vi "ILC Cyber Learning.vi"(6 "PID Cluster":T4={"L1 to L4 PID Cluster"={"L1 PID Gains"={"Kp"=0.005, "Kd"=0.5, "Ki"=0.0005}, "L2 PID Gains"={"Kp"=0.01, "Kd"=1.0, "Ki"=0.005}, "L3 PID Gains"={"Kp"=0.05, "Kd"=1.0, "Ki"=0.0005}, "L4 PID Gains"={"Kp"=0.1, "Kd"=0.1, "Ki"=0.0005}}, "Stage PID Cluster"={"Stage Z PID"={"Kp"=0.0005, "Kd"=0.001, "Ki"=0.0}, "Stage Y PID"={"Kp"=0.0003, "Kd"=0.01, "Ki"=0.0}, "Stage X PID"={"Kp"=0.0003, "Kd"=0.01, "Ki"=0.0}}, "OCT Z PID Gains"={"Kp"=0.0003, "Kd"=0.0001, "Ki"=0.01}}, 7 "Input RUY":T1, 8 "error in":errorcluster, 9 "Offset Home 2 RCM":dbl[](array[numeric])=[0.0, 0.0, 0.0, 0.0], 10 "Prev Posit Cluster":T3={"Prev L1 to L4 Posit"=[-0.5319, -0.035669172703475985, -2.0566170657346783, 0.9099264705882353], "Prev Stage Posit"=[6.002553885707208, 5.996566124542428, 5.995469940427586], "Prev OCT Z Posit"=-0.0}, 11 "FPGA VI Reference In":refnum<k20>) -> (0 "error out":errorcluster, 2 "Last Posit Cluster":T2={"Last L1 to L4 Posit"=[0.0, 0.0, 0.0, 0.0], "Last Stage Posit"=[6.0, 6.0, 6.0], "Last OCT Z Posit"=0.0}, 3 "FPGA VI Reference Out":refnum<k20>, 5 "Updated RUY":T1)   [LabVIEW 2016]
uses:
  <vilib>/Platform/TimedLoop/XDataNode/timing_clust.ctl
  <vilib>/Platform/TimedLoop/XDataNode/nitl_modes.ctl
  <vilib>/Platform/TimedLoop/XDataNode/wakeup.ctl
  Global Variables.vi
  <vilib>/platform/TimedLoop/XDataNode/XDataNode.xnode
  <vilib>/Platform/TimedLoop/XDataNode/XDNodeRunTimeDep.lvlib
panel:
  out "In Servo Loop":bool
  out "Loading Finished":bool
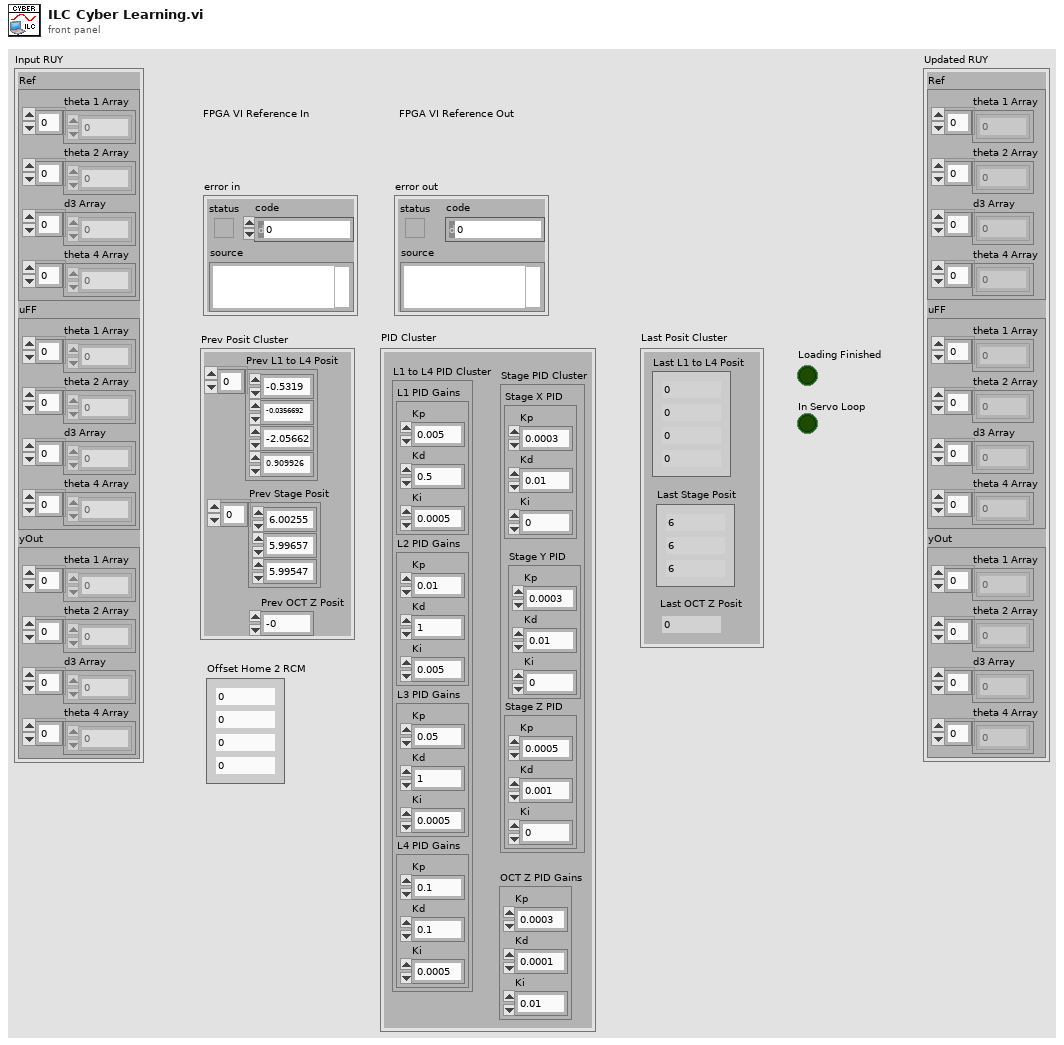
[diagram p1: front panel]
types:
  T1 = cluster{"Ref":cluster{"theta 1 Array":dbl[], "theta 2 Array":dbl[], "d3 Array":dbl[], "theta 4 Array":dbl[]}, "uFF":cluster{"theta 1 Array":dbl[], "theta 2 Array":dbl[], "d3 Array":dbl[], "theta 4 Array":dbl[]}, "yOut":cluster{"theta 1 Array":dbl[], "theta 2 Array":dbl[], "d3 Array":dbl[], "theta 4 Array":dbl[]}}
  T2 = cluster{"Last L1 to L4 Posit":dbl[], "Last Stage Posit":dbl[], "Last OCT Z Posit":dbl}
  T3 = cluster{"Prev L1 to L4 Posit":dbl[], "Prev Stage Posit":dbl[], "Prev OCT Z Posit":dbl}
  T4 = cluster{"L1 to L4 PID Cluster":cluster{"L1 PID Gains":cluster{"Kp":dbl, "Kd":dbl, "Ki":dbl}, "L2 PID Gains":cluster{"Kp":dbl, "Kd":dbl, "Ki":dbl}, "L3 PID Gains":cluster{"Kp":dbl, "Kd":dbl, "Ki":dbl}, "L4 PID Gains":cluster{"Kp":dbl, "Kd":dbl, "Ki":dbl}}, "Stage PID Cluster":cluster{"Stage Z PID":cluster{"Kp":dbl, "Kd":dbl, "Ki":dbl}, "Stage Y PID":cluster{"Kp":dbl, "Kd":dbl, "Ki":dbl}, "Stage X PID":cluster{"Kp":dbl, "Kd":dbl, "Ki":dbl}}, "OCT Z PID Gains":cluster{"Kp":dbl, "Kd":dbl, "Ki":dbl}}
  T5 = cluster{"Stop Vacuum":bool, "Vacuum Force":i8, "Max Limit [mmHg]":dbl, "Slide in":i8, "Irrigation?":bool}
  T6 = typedef "XDNodeRunTimeDep.lvlib/timing_clust.ctl" = cluster{"Expected End [f-1]":u64, "Actual End [f-1]":u64, "Finished Late? [f-1]":bool, "Expected End [i-1]":u64, "Actual End [i-1]":u64, "Finished Late? [i-1]":bool, "Expected Start [i]":u64, "Actual Start [i]":u64, "Expected Start [f]":u64, "Actual Start [f]":u64, "Source Name":string, "Structure Name":string, "Period":i64, "Deadline":i64, "Offset":i64, "Start":i64, "Priority":i32, "Timeout":i32, "Mode":T7, "Wakeup Reason":T8, "Error":errorcluster, "Source Type":string, "Secondary Source Type":string, "Global End Time":u64, "Global Start Time":u64, "Frame Duration":u64, "Iteration Duration":u64, "Assigned CPU":i32, "I/O Scan Engine Mode":u32}
  T7 = typedef "XDNodeRunTimeDep.lvlib/nitl_modes.ctl" = enum32{"No Change", "Process missed periods, maintain original phase", "Discard missed periods, maintain original phase", "Process missed periods, ignore original phase", "Discard missed periods, ignore original phase"}
  T8 = typedef "XDNodeRunTimeDep.lvlib/wakeup.ctl" = enum32{"Normal", "Aborted", "Asynchronous wakeup", "Timing source error", "Timed loop error", "Timeout"}
  T9 = cluster{"L1 PID Gains":cluster{"Kp":dbl, "Kd":dbl, "Ki":dbl}, "L2 PID Gains":cluster{"Kp":dbl, "Kd":dbl, "Ki":dbl}, "L3 PID Gains":cluster{"Kp":dbl, "Kd":dbl, "Ki":dbl}, "L4 PID Gains":cluster{"Kp":dbl, "Kd":dbl, "Ki":dbl}}
  T10 = cluster{"Stage Z PID":cluster{"Kp":dbl, "Kd":dbl, "Ki":dbl}, "Stage Y PID":cluster{"Kp":dbl, "Kd":dbl, "Ki":dbl}, "Stage X PID":cluster{"Kp":dbl, "Kd":dbl, "Ki":dbl}}
  T11 = cluster{"Accurus button":bool[], "Accurus engaged?":bool, "Vacuum Force":i32, "Accurus Ch. A Vout":dbl, "Accurus Ch. B Vout":dbl, "Irrigation engaged?":bool}
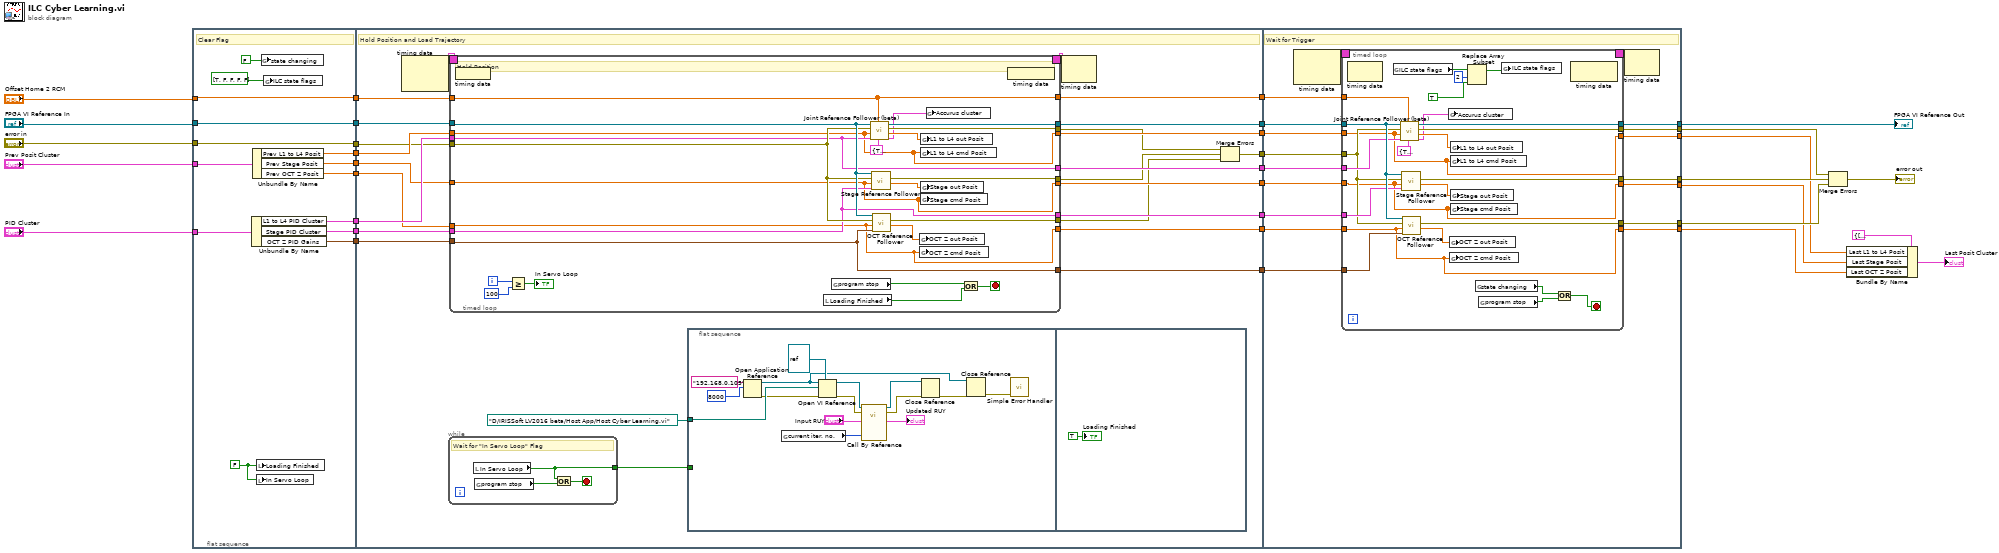
[diagram p0: block diagram]
diagram:
  n1 = flat-sequence {
    tunnel: [w46] -> w33
    tunnel: "FPGA VI Reference In" -> [w46]
    tunnel: [w45] -> w31
    tunnel: "error in" -> [w45]
    tunnel: "Prev Posit Cluster" -> [w44]
    tunnel: "PID Cluster" -> [w43]
    tunnel: [w42] -> w29
    tunnel: [w41] -> w28
    tunnel: "Offset Home 2 RCM" -> [w40]
    tunnel: [w40] -> w26
    tunnel: [w39] -> w23
    tunnel: [w38] -> w22
    tunnel: [w37] -> w21
    tunnel: [w36] -> w20
    tunnel: w33 -> [w60]
    tunnel: w31 -> [w55]
    tunnel: w29 -> [w57]
    tunnel: w28 -> [w56]
    tunnel: w26 -> [w61]
    tunnel: w23 -> [w59]
    tunnel: w22 -> [w54]
    tunnel: w21 -> [w53]
    tunnel: w20 -> [w58]
    tunnel: [w72] -> w9
    tunnel: [w71] -> w8
    tunnel: [w70] -> w7
    tunnel: [w69] -> w6
    tunnel: [w68] -> w5
    tunnel: [w67] -> w4
    tunnel: [w66] -> w3
    tunnel: [w65] -> w2
    tunnel: [w49] -> w1
    tunnel: w9 -> [w135]
    tunnel: [w134] -> w18
    tunnel: [w133] -> w17
    tunnel: [w132] -> w16
    tunnel: w8 -> [w131]
    tunnel: w7 -> [w130]
    tunnel: w6 -> [w129]
    tunnel: w5 -> [w128]
    tunnel: w4 -> [w127]
    tunnel: w3 -> [w126]
    tunnel: w2 -> [w125]
    tunnel: [w124] -> w14
    tunnel: [w123] -> w13
    tunnel: [w122] -> w12
    tunnel: [w121] -> w10
    tunnel: w1 -> [w120]
    frame #0 {
      w35 = FALSE ("Loading Finished")
      # "Clear Flag"
      n2 = Unbundle By Name(w43) -> ("L1 to L4 PID Cluster"=w41:T9, "Stage PID Cluster"=w42:T10, "OCT Z PID Gains"=w36:cluster{"Kp":dbl, "Kd":dbl, "Ki":dbl})
      n3 = Unbundle By Name(w44) -> ("Prev L1 to L4 Posit"=w39:dbl[], "Prev Stage Posit"=w38:dbl[], "Prev OCT Z Posit"=w37:dbl)
      n4 = local write "Loading Finished"(w35) -> ()
      n5 = local write "In Servo Loop"(w35) -> ()
      n6 = global write "Global Variables.vi" "state changing"(FALSE ("state changing")) -> ()
      n7 = global write "Global Variables.vi" "ILC state flags"(bool[] [TRUE, FALSE, FALSE, FALSE, FALSE]) -> ()
    }
    frame #1 {
      # "Hold Position and Load Trajectory"
      n8 = node-c288() -> (w64:T6)  [unwired: 2 in]
      n9 = while {
        tunnel: [w74] -> w62
        stop <- w75 stop-if-true
        # "Wait for \"In Servo Loop\" Flag"
        n10 = local read "In Servo Loop"() -> (w74:bool)
        n11 = global read "Global Variables.vi" "program stop"() -> (w73:bool)
        n12 = Or(x=w74, y=w73) -> (x .or. y?=w75:bool)
      }
      n13 = timed-loop {
        timing: w64 -> [_]
        timing-out: [_] -> w63
        tunnel: w59 -> [w94]
        tunnel: w54 -> [w93]
        tunnel: w57 -> [w100]
        tunnel: w56 -> [w101]
        tunnel: w55 -> [w111]
        tunnel: w60 -> [w112]
        tunnel: w61 -> [w107]
        tunnel: w53 -> [w92]
        tunnel: w58 -> [w102]
        tunnel: [w94] -> w70
        tunnel: [w93] -> w69
        tunnel: [w92] -> w68
        tunnel: [w107] -> w71
        tunnel: [w106] -> w72
        tunnel: [w105] -> w52
        tunnel: [w104] -> w51
        tunnel: [w103] -> w50
        tunnel: [w102] -> w67
        tunnel: [w101] -> w66
        tunnel: [w100] -> w65
        i -> [w99]
        stop <- w115 stop-if-true
        # "Hold Position"
        n14 = node-c288 ("Output Node")() -> ()  [unwired: 1 in]
        n15 = Greater Or Equal?(x=w99, y=100) -> (x >= y?=→"In Servo Loop":bool)
        n16 = local read "Loading Finished"() -> (w114:bool)
        n17 = global read "Global Variables.vi" "program stop"() -> (w113:bool)
        n18 = call "Joint Reference Follower (beta).vi"("Accurus Ctrl Cluster"=T5 {"Stop Vacuum"=TRUE, "Vacuum Force"=0, "Max Limit [mmHg]"=600.0, "Slide in"=0, "Irrigation?"=TRUE}, "Offset Home2RCM [deg/mm]"=w107, "PID Ctrl Cluster"=w101, "Ref Array [deg/mm]"=w94, "error in"=w111, "FPGA VI Reference In"=w112) -> ("Accurus Output Cluster"=w95:T11, "Output Posit Array [deg/mm]"=w110:dbl[], "error out"=w105:errorcluster, "FPGA VI Reference Out"=w106:refnum<k20>)  [unwired: 2 in]
        n19 = call "Stage Reference Follower.vi"("Stage PID Cluster"=w100, "Stage cmd Posit [mm]"=w93, "error in"=w111, "FPGA VI Reference In"=w112) -> ("Stage out Posit [mm]"=w109:dbl[], "error out"=w104:errorcluster)  [unwired: 5 in, 1 out]
        n20 = call "OCT Reference Follower.vi"("OCT Z PID Gains"=w102, "OCT  Z cmd Posit [mm]"=w92, "error in"=w111, "FPGA VI Reference In"=w112) -> ("OCT  Z out Posit [mm]"=w108:dbl, "error out"=w103:errorcluster)  [unwired: 5 in, 1 out]
        n21 = global write "Global Variables.vi" "OCT Z out Posit"(w108) -> ()
        n22 = global write "Global Variables.vi" "OCT Z cmd Posit"(w92) -> ()
        n23 = global write "Global Variables.vi" "L1 to L4 out Posit"(w110) -> ()
        n24 = global write "Global Variables.vi" "L1 to L4 cmd Posit"(w94) -> ()
        n25 = global write "Global Variables.vi" "Stage out Posit"(w109) -> ()
        n26 = global write "Global Variables.vi" "Stage cmd Posit"(w93) -> ()
        n27 = global write "Global Variables.vi" "Accurus cluster"(w95) -> ()
        n28 = Or(x=w113, y=w114) -> (x .or. y?=w115:bool)
        n29 = node-c288() -> ()  [unwired: 1 out]
      }
      n30 = flat-sequence {
        tunnel: w62 -> [_]
        tunnel: path "D:/IRISSoft LV2016 beta/Host App/Host Cyber Learning.vi" ("vi path") -> [w82]
        frame #0 {
          n31 = Open Application Reference(10:u16 8000 ("port number or service name (3363)"), 11:"192.168.0.105" ("machine name (\"\":  open local reference)")) -> (0:w79:errorcluster, 3:w84:refnum<vi>)  [unwired: 2 in]
          n32 = global read "Global Variables.vi" "current iter. no."() -> (w76:u16)
          n33 = Open VI Reference(type specifier VI Refnum (for type only)=refnum<vi> refnum, application reference (local)=w84, vi path=w82, error in (no error)=w79) -> (vi reference=w86:refnum<vi>, error out=w81:errorcluster)  [unwired: 2 in]
          n34 = call-by-ref "?"(reference=w86, error in=w81, "Curr Iter No"=w76, "Input RUY"="Input RUY") -> (reference out=w87:refnum<vi>, error out=w80:errorcluster, "Updated RUY"=→"Updated RUY":T1)  [unwired: 9 in]
          n35 = Close Reference(reference=w87, error in (no error)=w80) -> (error out=w83:errorcluster)
          n36 = Close Reference(reference=w84, error in (no error)=w83) -> (error out=w78:errorcluster)
          n37 = call <vilib>:"Simple Error Handler.vi"("error in (no error)"=w78) -> ()  [unwired: 4 in, 5 out]
        }
        frame #1 {
          "Loading Finished" <- TRUE ("Loading Finished")
        }
      }
      n38 = node-c288(w63) -> ()  [unwired: 1 out]
      n39 = Merge Errors(w52, w51, w50) -> (w49:errorcluster)
    }
    frame #2 {
      # "Wait for Trigger"
      n40 = node-c288() -> (w137:T6)  [unwired: 2 in]
      n41 = timed-loop {
        timing: w137 -> [_]
        timing-out: [_] -> w136
        tunnel: w135 -> [w155]
        tunnel: [w154] -> w133
        tunnel: [w153] -> w134
        tunnel: [w152] -> w132
        tunnel: w131 -> [w151]
        tunnel: w130 -> [w140]
        tunnel: w129 -> [w139]
        tunnel: w128 -> [w138]
        tunnel: w127 -> [w150]
        tunnel: w126 -> [w149]
        tunnel: w125 -> [w148]
        tunnel: [w140] -> w124
        tunnel: [w139] -> w123
        tunnel: [w138] -> w122
        tunnel: [w144] -> w121
        tunnel: w120 -> [w143]
        stop <- w162 stop-if-true
        n42 = node-c288() -> ()  [unwired: 1 in, 1 out]
        n43 = global read "Global Variables.vi" "ILC state flags"() -> (w159:bool[])
        n44 = call "Joint Reference Follower (beta).vi"("Accurus Ctrl Cluster"=T5 {"Stop Vacuum"=TRUE, "Vacuum Force"=0, "Max Limit [mmHg]"=600.0, "Slide in"=0, "Irrigation?"=TRUE}, "Offset Home2RCM [deg/mm]"=w151, "PID Ctrl Cluster"=w149, "Ref Array [deg/mm]"=w140, "error in"=w143, "FPGA VI Reference In"=w155) -> ("Accurus Output Cluster"=w141:T11, "Output Posit Array [deg/mm]"=w147:dbl[], "error out"=w154:errorcluster, "FPGA VI Reference Out"=w144:refnum<k20>)  [unwired: 2 in]
        n45 = call "Stage Reference Follower.vi"("Stage PID Cluster"=w148, "Stage cmd Posit [mm]"=w139, "error in"=w143, "FPGA VI Reference In"=w155) -> ("Stage out Posit [mm]"=w146:dbl[], "error out"=w153:errorcluster)  [unwired: 5 in, 1 out]
        n46 = call "OCT Reference Follower.vi"("OCT Z PID Gains"=w150, "OCT  Z cmd Posit [mm]"=w138, "error in"=w143, "FPGA VI Reference In"=w155) -> ("OCT  Z out Posit [mm]"=w145:dbl, "error out"=w152:errorcluster)  [unwired: 5 in, 1 out]
        n47 = global write "Global Variables.vi" "Accurus cluster"(w141) -> ()
        n48 = global write "Global Variables.vi" "OCT Z out Posit"(w145) -> ()
        n49 = global write "Global Variables.vi" "OCT Z cmd Posit"(w138) -> ()
        n50 = global write "Global Variables.vi" "L1 to L4 out Posit"(w147) -> ()
        n51 = global write "Global Variables.vi" "L1 to L4 cmd Posit"(w140) -> ()
        n52 = global write "Global Variables.vi" "Stage out Posit"(w146) -> ()
        n53 = global write "Global Variables.vi" "Stage cmd Posit"(w139) -> ()
        n54 = Replace Array Subset(array=w159, new element=TRUE ("new element/subarray"), index=2) -> (w158:bool[])
        n55 = global read "Global Variables.vi" "state changing"() -> (w161:bool)
        n56 = global read "Global Variables.vi" "program stop"() -> (w160:bool)
        n57 = global write "Global Variables.vi" "ILC state flags"(w158) -> ()
        n58 = Or(x=w161, y=w160) -> (x .or. y?=w162:bool)
        n59 = node-c288() -> ()  [unwired: 1 in, 1 out]
      }
      n60 = node-c288(w136) -> ()  [unwired: 1 out]
    }
  }
  n61 = Merge Errors(w17, w18, w16) -> (→"error out":errorcluster)
  n62 = Bundle By Name(cluster=T2 {"Last L1 to L4 Posit"=[0.0, 0.0, 0.0, 0.0], "Last Stage Posit"=[6.0, 6.0, 6.0], "Last OCT Z Posit"=0.0} ("Last Posit Cluster 2"), "Last L1 to L4 Posit"=w14, "Last Stage Posit"=w13, "Last OCT Z Posit"=w12) -> (→"Last Posit Cluster":T2)
  "FPGA VI Reference Out" <- w10
